vi "DisplayBottomColorVer_DP_2.0.vi"(3 "WFGraph Ref.":refnum<vi>, 4 "Scale Arr Refnum":refnum<vi>, 5 "Y Ref. Output":refnum<vi>[](array[refnum])) -> ()   [LabVIEW 2012]
doc: "The color of tex inside the \"Display control\" is set. The color of tex is match to the corresponding \"plot color\" in the XY graph. \nThe Y scale index(L or R) of plot is set based on the \"Scale\" array in the \"Display control\""
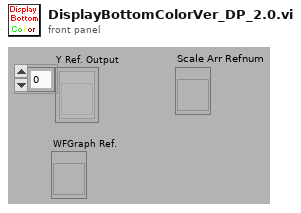
[diagram p1: front panel]
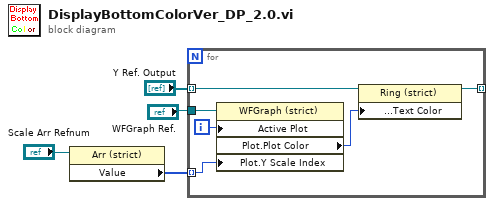
[diagram p0: block diagram]
diagram:
  n1 = property class="Arr (strict)"(reference="Scale Arr Refnum") -> ("Value"=w1:u16[])  [unwired: 1 in, 2 out]
  n2 = for {
    tunnel: "WFGraph Ref." -> [w10]
    tunnel: "Y Ref. Output" -> [w8] mode=indexing
    tunnel: [w7] -> _ mode=indexing
    tunnel: w1 -> [w5] mode=indexing
    i -> [w9]
    n3 = property class="WFGraph (strict)"(reference=w10, "Active Plot"=w9, "Plot.Y Scale Index"=w5) -> ("Plot.Plot Color"=w6:u32)  [unwired: 1 in, 2 out]
    n4 = property class="Ring (strict)"(reference=w8, "Named Numeric Colors:Text Color"=w6) -> (reference out=w7:refnum<vi>)  [unwired: 1 in, 1 out]
  }
